vi "LCDWriteBitmap.vi"(5 "ySize":i32, 6 "Bitmap":u8[](array[numeric]), 7 "xSize":i32, 8 "error in (no error)":errorcluster, 9 "ypos":i32, 10 "xpos":i32, 11 "Device In":u64) -> (0 "error out":errorcluster, 3 "Device Out":u64)   [LabVIEW 2012, in "Phidget LCD.lvlib"]
doc: "${WriteBitmap:Header}"
uses:
  <instrlib>/Phidgets/Phidget LCD/Phidget LCD.lvlib
  <instrlib>/Phidgets/Phidget Common/Phidget Common.lvlib
  phidget22.dll
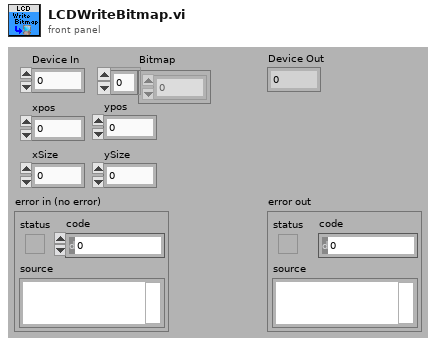
[diagram p1: front panel]
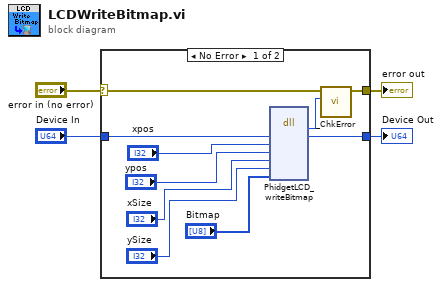
[diagram p0: block diagram]
diagram:
  n1 = case shown="No Error" "error in (no error)" {
    selector: "error in (no error)" -> [w12 w16]
    tunnel: [w11 w16] -> w3
    tunnel: "Device In" -> [w14 w15]
    tunnel: [w13 w15] -> w1
    frame No Error {
      n2 = dll-call lib="phidget22.*" fn="PhidgetLCD_writeBitmap"("phid"=w14, "xpos"="xpos", "ypos"="ypos", "xSize"="xSize", "ySize"="ySize", "bitmap"="Bitmap") -> ("return type"=w10:i32, "phid"=w13:u64)  [unwired: 8 in, 2 out]
      n3 = call <instrlib>:"_ChkError.vi"("Return Code"=w10, "error in (no error)"=w12) -> ("error out"=w11:errorcluster)  [unwired: 9 in]
    }
    frame Error {
    }
  }
  "error out" <- w3
  "Device Out" <- w1
